vi "Bella_MagSpec_simple_file_reader.vi"() -> ()   [LabVIEW 2011]
uses:
  <vilib>/vision/NI_Vision_Development_Module.lvlib
panel:
  in  "File Path":path
  out "error out 2":errorcluster
  out "error out":errorcluster
  out "Momentum 14":dbl=2.780793 caption="Momentum (GeV/c)" min=0.0 max=0.0 format="%#.1f"
  out "Momentum 13":dbl=2.780793 caption="Momentum (GeV/c)" min=0.0 max=0.0 format="%#.1f"
  out "Momentum 12":dbl=2.780793 caption="Momentum (GeV/c)" min=0.0 max=0.0 format="%#.1f"
  out "Momentum 11":dbl=2.780793 caption="Momentum (GeV/c)" min=0.0 max=0.0 format="%#.1f"
  out "Momentum 10":dbl=2.780793 caption="Momentum (GeV/c)" min=0.0 max=0.0 format="%#.1f"
  out "Momentum 9":dbl=2.780793 caption="Momentum (GeV/c)" min=0.0 max=0.0 format="%#.1f"
  out "Momentum 8":dbl=2.780793 caption="Momentum (GeV/c)" min=0.0 max=0.0 format="%#.1f"
  out "Momentum 7":dbl=2.780793 caption="Momentum (GeV/c)" min=0.0 max=0.0 format="%#.1f"
  out "Momentum 6":dbl=2.780793 caption="Momentum (GeV/c)" min=0.0 max=0.0 format="%#.1f"
  out "Momentum 5":dbl=2.780793 caption="Momentum (GeV/c)" min=0.0 max=0.0 format="%#.1f"
  out "Momentum 4":dbl=2.780793 caption="Momentum (GeV/c)" min=0.0 max=0.0 format="%#.1f"
  out "Momentum 3":dbl=2.780793 caption="Momentum (GeV/c)" min=0.0 max=0.0 format="%#.1f"
  out "Momentum 2":dbl=2.780793 caption="Momentum (GeV/c)" min=0.0 max=0.0 format="%#.1f"
  out "Momentum 1":dbl=2.780793 caption="Momentum (GeV/c)" min=0.0 max=0.0 format="%#.1f"
  out "image::13":T1(plugin-control) caption="M1 Cam"
  out "image::12":T1(plugin-control) caption="M1 Cam"
  out "image::11":T1(plugin-control) caption="M1 Cam"
  out "image::10":T1(plugin-control) caption="M1 Cam"
  out "image::9":T1(plugin-control) caption="M1 Cam"
  out "image::8":T1(plugin-control) caption="M1 Cam"
  out "image::7":T1(plugin-control) caption="M1 Cam"
  out "image::6":T1(plugin-control) caption="M1 Cam"
  out "image::5":T1(plugin-control) caption="M1 Cam"
  out "flipped2":T1(plugin-control) caption="M1 Cam"
  out "flipped1":T1(plugin-control) caption="M1 Cam"
  out "image::4":T1(plugin-control) caption="M1 Cam"
  out "image::3":T1(plugin-control) caption="M1 Cam"
  out "image::2":T1(plugin-control) caption="M1 Cam"
  out "image::1":T1(plugin-control) caption="M1 Cam"
  in  "Field::14":dbl=2.780793 caption="Magnetic Field (mT)" min=0.0 max=0.0 format="%_4f"
  out "Boolean":bool
  # "MeV/c"
  # "MeV/c"
  # "MeV/c"
  # "MeV/c"
  # "H:\\data\\Y2013\\03-Mar\\13_0311\\scans\\Scan011\\MagSpecA\\Scan011_MagSpecA_166.png"
  # "H:\\data\\Y2013\\03-Mar\\13_0311\\scans\\Scan011\\MagSpecA\\Scan011_MagSpecA_219.png"
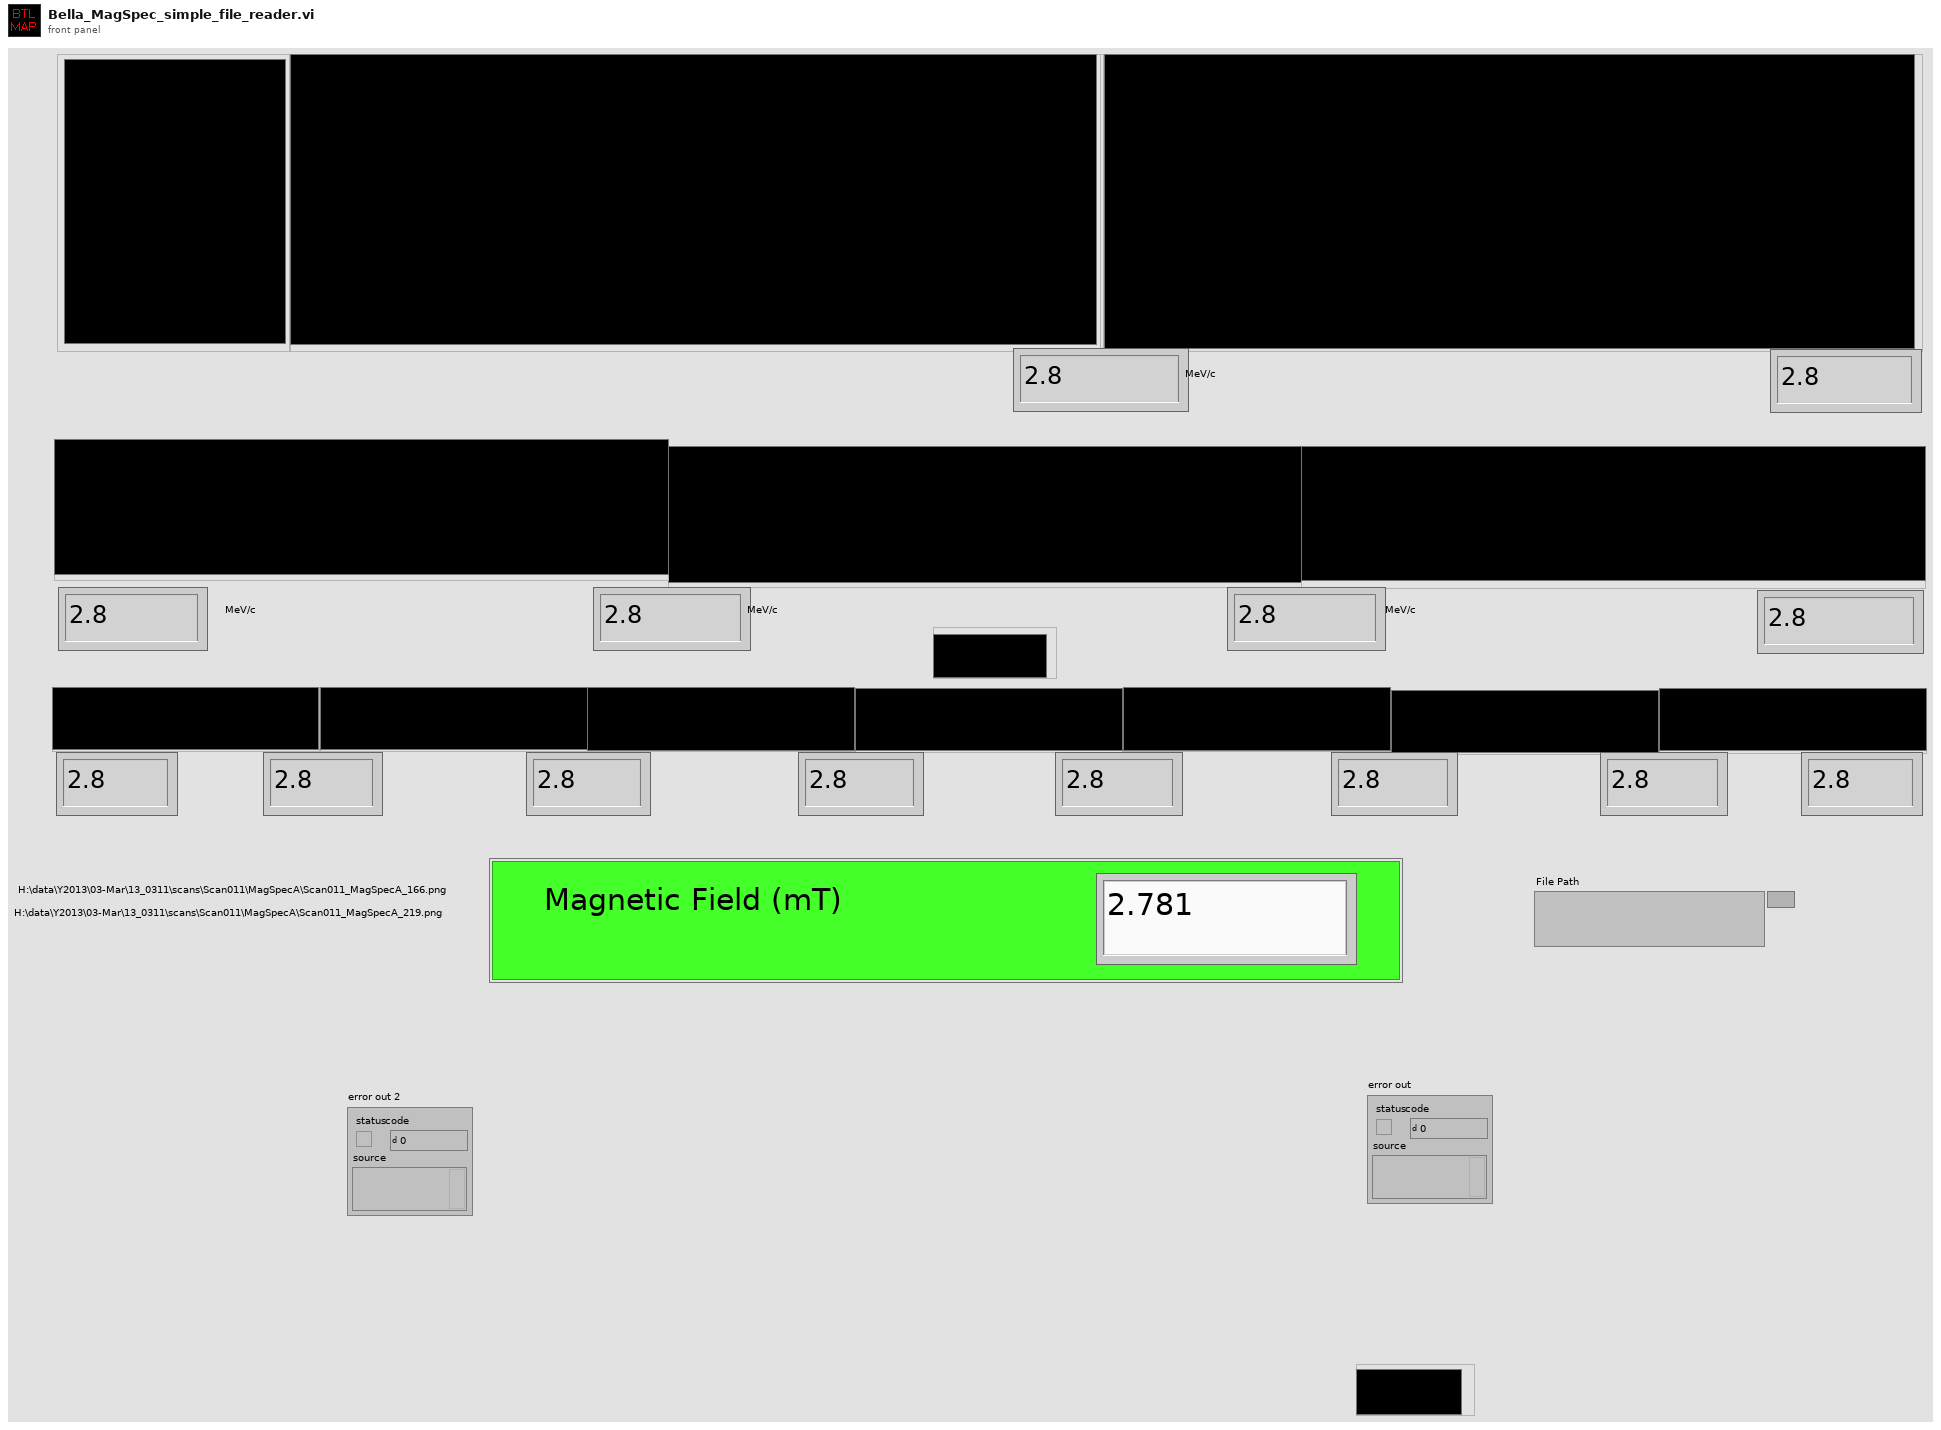
[diagram p1: front panel]
types:
  T1 = typedef "IMAQ Image.ctl" = refnum<image>
  T2 = typedef "Image Type" = u32
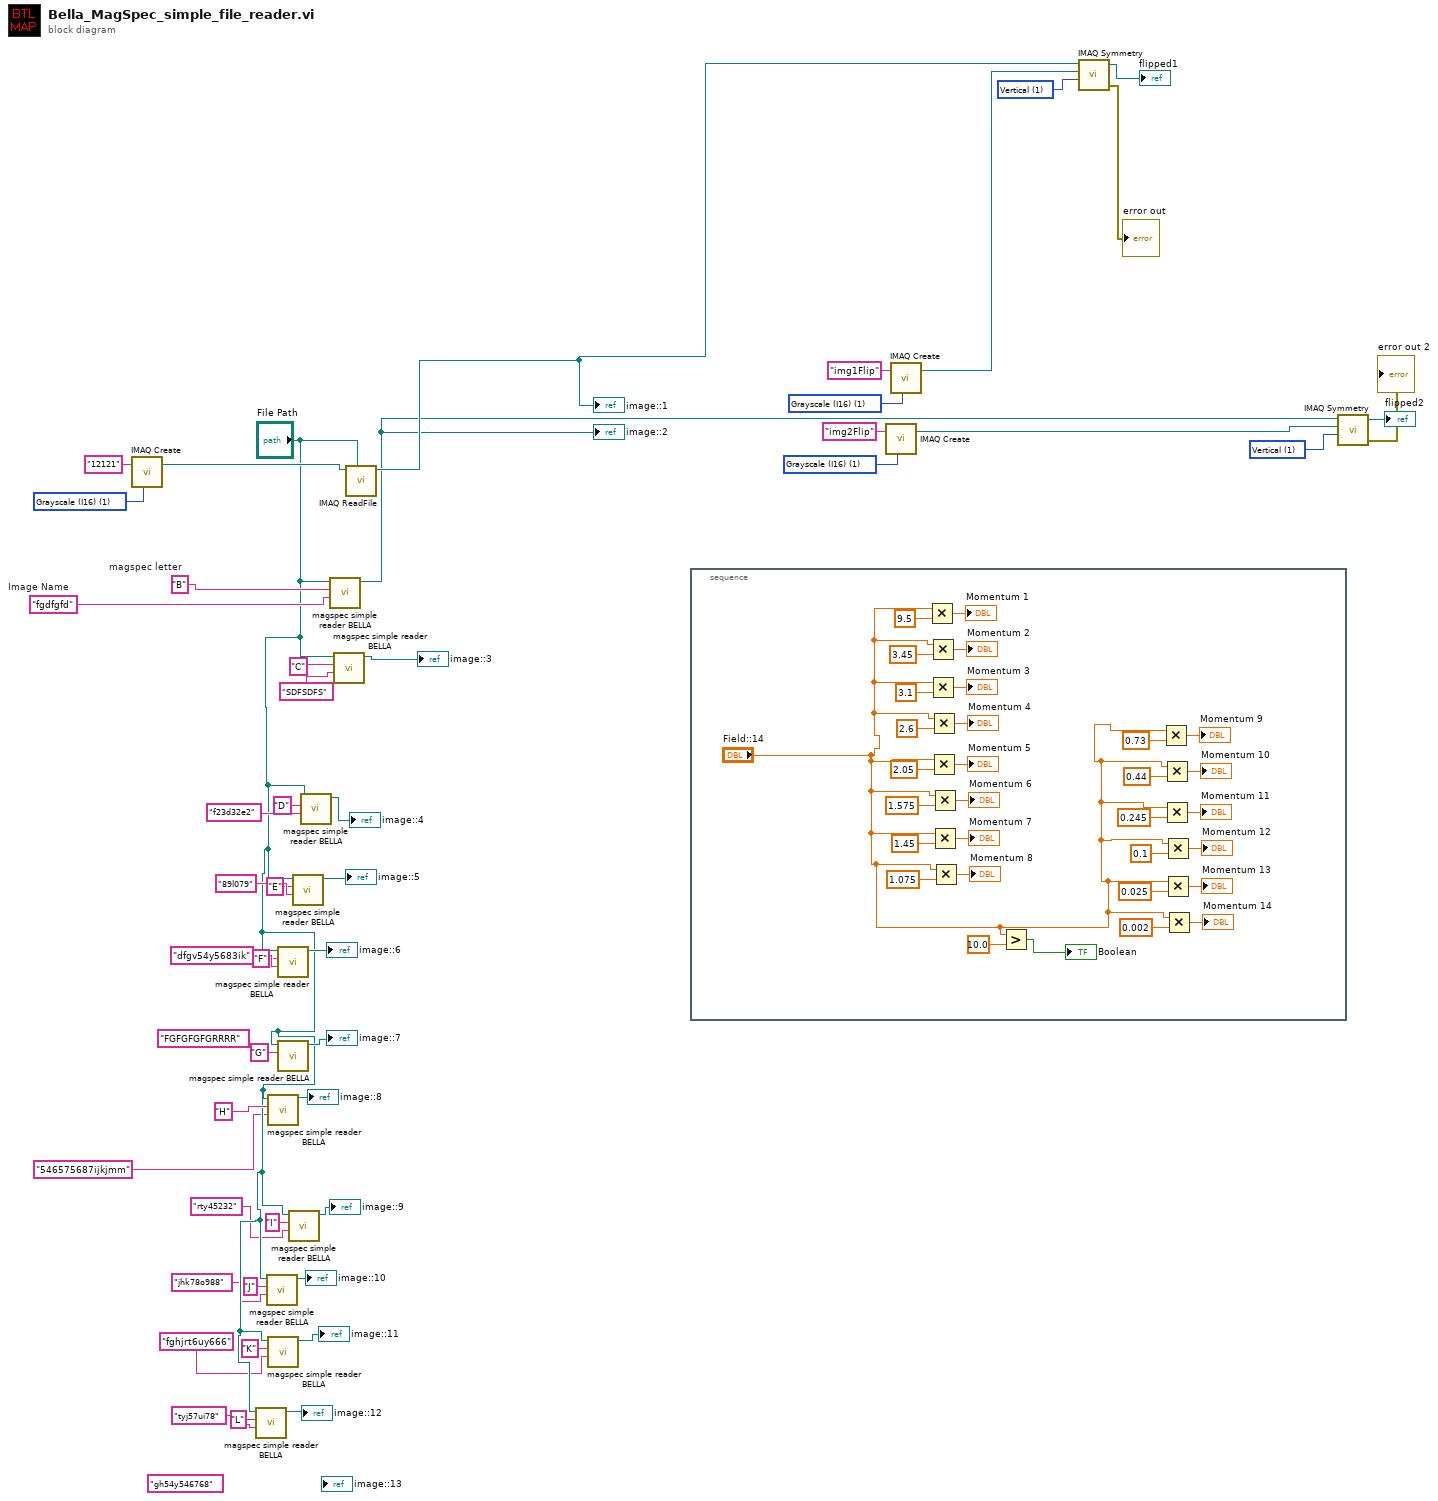
[diagram p0: block diagram]
diagram:
  w32 = "B"  # magspec letter
  w37 = u32 1 items=["Horizontal", "Vertical", "Central", "1st Diagonal", "2nd Diagonal"] ("Type of Symmetry")
  w40 = u32 1 items=["Horizontal", "Vertical", "Central", "1st Diagonal", "2nd Diagonal"] ("Type of Symmetry")
  (unwired) "gh54y546768" ("Image Name")
  (unwired) "FGFGFGFGRRRR" ("Image Name")
  w42 = "fgdfgfd"  # Image Name
  w44 = T2 1 items=["Grayscale (U8)", "Grayscale (I16)", "Grayscale (SGL)", "Complex (CSG)", "RGB (U32)", "HSL (U32)", "RGB (U64)", "Grayscale (U16)"] ("Image Type")
  w47 = T2 1 items=["Grayscale (U8)", "Grayscale (I16)", "Grayscale (SGL)", "Complex (CSG)", "RGB (U32)", "HSL (U32)", "RGB (U64)", "Grayscale (U16)"] ("Image Type")
  w48 = T2 1 items=["Grayscale (U8)", "Grayscale (I16)", "Grayscale (SGL)", "Complex (CSG)", "RGB (U32)", "HSL (U32)", "RGB (U64)", "Grayscale (U16)"] ("Image Type")
  n1 = call "IMAQ Create"("Image Name"="12121", "Image Type"=w44) -> ("New Image"=w34:T1)  [unwired: 3 in, 1 out]
  n2 = call "magspec simple reader BELLA.vi"("Image Name"="tyj57ui78", "magspec letter"="L", "File Path"="File Path") -> ("Refnum out"=→"image::12":T1)  [unwired: 8 in]
  n3 = call "magspec simple reader BELLA.vi"("Image Name"="jhk78o988", "magspec letter"="J", "File Path"="File Path") -> ("Refnum out"=→"image::10":T1)  [unwired: 8 in]
  n4 = call "magspec simple reader BELLA.vi"("Image Name"="546575687ijkjmm", "magspec letter"="H", "File Path"="File Path") -> ("Refnum out"=→"image::8":T1)  [unwired: 8 in]
  n5 = call "magspec simple reader BELLA.vi"("Image Name"="fghjrt6uy666", "magspec letter"="K", "File Path"="File Path") -> ("Refnum out"=→"image::11":T1)  [unwired: 8 in]
  n6 = call "magspec simple reader BELLA.vi"("Image Name"="dfgv54y5683ik", "magspec letter"="F", "File Path"="File Path") -> ("Refnum out"=→"image::6":T1)  [unwired: 8 in]
  n7 = call "magspec simple reader BELLA.vi"("magspec letter"="G", "File Path"="File Path") -> ("Refnum out"=→"image::7":T1)  [unwired: 9 in]
  n8 = call "magspec simple reader BELLA.vi"("Image Name"="rty45232", "magspec letter"="I", "File Path"="File Path") -> ("Refnum out"=→"image::9":T1)  [unwired: 8 in]
  n9 = call "magspec simple reader BELLA.vi"("Image Name"="89l079", "magspec letter"="E", "File Path"="File Path") -> ("Refnum out"=→"image::5":T1)  [unwired: 8 in]
  n10 = call "magspec simple reader BELLA.vi"("Image Name"="f23d32e2", "magspec letter"="D", "File Path"="File Path") -> ("Refnum out"=→"image::4":T1)  [unwired: 8 in]
  n11 = call "magspec simple reader BELLA.vi"("Image Name"=w42, "magspec letter"=w32, "File Path"="File Path") -> ("Refnum out"=w33:T1)  [unwired: 8 in]
  "image::2" <- w33
  n12 = call "magspec simple reader BELLA.vi"("Image Name"="SDFSDFS" ("magspec letter"), "magspec letter"="C" ("Image Name"), "File Path"="File Path") -> ("Refnum out"=→"image::3":T1)  [unwired: 8 in]
  n13 = call "IMAQ ReadFile"("File Path"="File Path", "Image"=w34) -> ("Image Out"=w35:T1)  [unwired: 5 in, 4 out]
  "image::1" <- w35
  n14 = stacked-sequence {
    frame #0 {
      n15 = Multiply(x="Field::14", y=9.5) -> (x*y=→"Momentum 1":dbl)
      n16 = Multiply(x="Field::14", y=3.45) -> (x*y=→"Momentum 2":dbl)
      n17 = Multiply(x="Field::14", y=3.1) -> (x*y=→"Momentum 3":dbl)
      n18 = Multiply(x="Field::14", y=2.6) -> (x*y=→"Momentum 4":dbl)
      n19 = Multiply(x="Field::14", y=2.05) -> (x*y=→"Momentum 5":dbl)
      n20 = Multiply(x="Field::14", y=1.575) -> (x*y=→"Momentum 6":dbl)
      n21 = Multiply(x="Field::14", y=1.45) -> (x*y=→"Momentum 7":dbl)
      n22 = Multiply(x="Field::14", y=1.075) -> (x*y=→"Momentum 8":dbl)
      n23 = Greater?(x="Field::14", y=10.0) -> (0:→"Boolean":bool)
      n24 = Multiply(x="Field::14", y=0.73) -> (x*y=→"Momentum 9":dbl)
      n25 = Multiply(x="Field::14", y=0.44) -> (x*y=→"Momentum 10":dbl)
      n26 = Multiply(x="Field::14", y=0.245) -> (x*y=→"Momentum 11":dbl)
      n27 = Multiply(x="Field::14", y=0.1) -> (x*y=→"Momentum 12":dbl)
      n28 = Multiply(x="Field::14", y=0.025) -> (x*y=→"Momentum 13":dbl)
      n29 = Multiply(x="Field::14", y=0.002) -> (x*y=→"Momentum 14":dbl)
    }
  }
  n30 = call "IMAQ Create"("Image Name"="img2Flip", "Image Type"=w47) -> ("New Image"=w45:T1)  [unwired: 3 in, 1 out]
  n31 = call "IMAQ Create"("Image Name"="img1Flip", "Image Type"=w48) -> ("New Image"=w7:T1)  [unwired: 3 in, 1 out]
  n32 = call "IMAQ Symmetry"("Type of Symmetry"=w40, "Image Dst"=w7, "Image Src"=w35) -> ("error out"=→"error out":errorcluster, "Image Dst Out"=→"flipped1":T1)  [unwired: 2 in]
  n33 = call "IMAQ Symmetry"("Type of Symmetry"=w37, "Image Dst"=w45, "Image Src"=w33) -> ("error out"=→"error out 2":errorcluster, "Image Dst Out"=→"flipped2":T1)  [unwired: 2 in]
